vi "RangeSearch.vi"() -> ()   [LabVIEW 2019]
panel:
  in  "Start":bool
  in  "File Type":bool
  in  "stop":bool
  out "RPM Output":dbl
  out "Closest Range":dbl
  out "Array Index":dbl
  out "Search Value":dbl
  in  "Range":dbl(slide) scale=9.0..14.0
  out "Fractional Index":dbl
  out "Searched Part of 2D Array":dbl[](array[numeric])
  out "Input File":string
  out "Output Array":dbl[][](array[numeric])
  # "CSV Delimited"
  # "Tab Delimited"
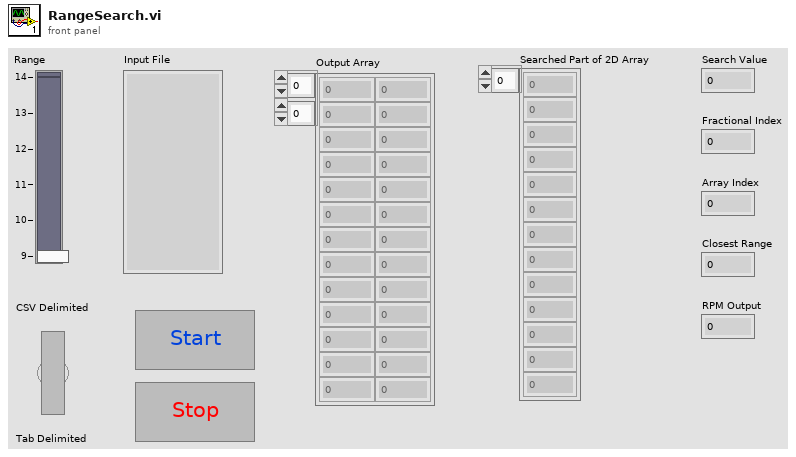
[diagram p1: front panel]
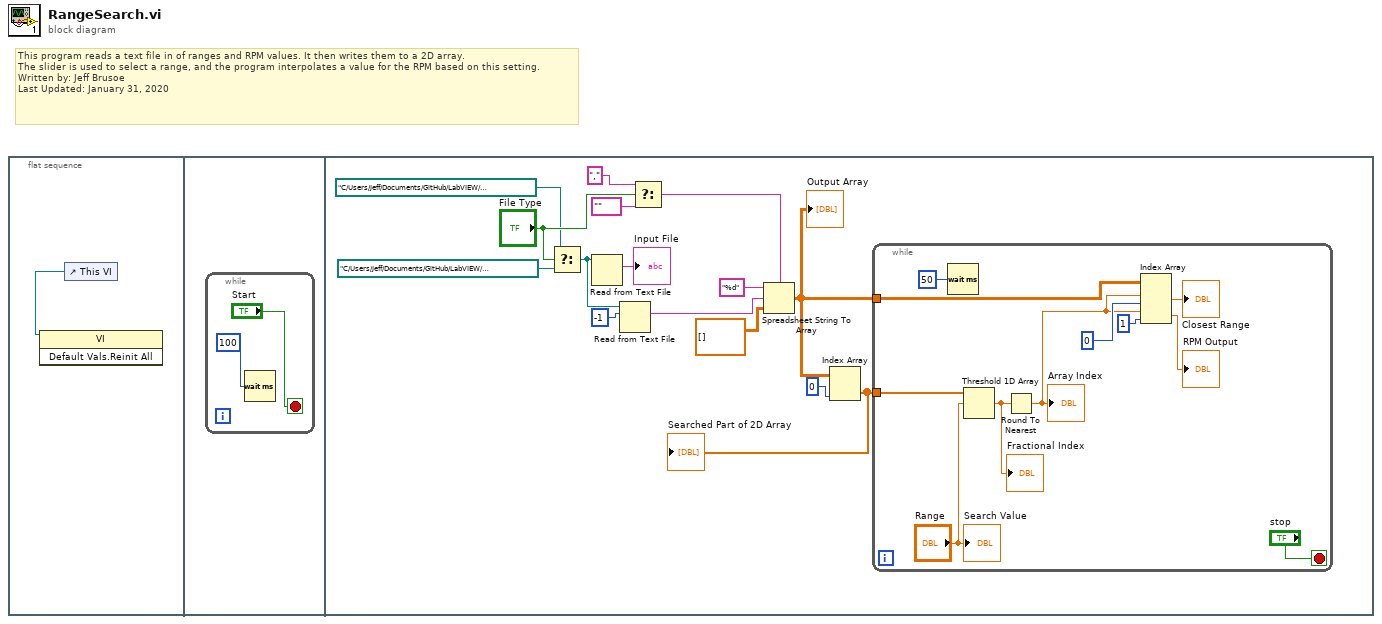
[diagram p0: block diagram]
diagram:
  # "This program reads a text file in of ranges and RPM values. It then writes them to a 2D array.\nThe slider is used to select a range, and the program interpolates a value for the RPM based on this setting.\nWritten by: Jeff Brusoe\nLast Updated: January 31, 2020"
  n1 = flat-sequence {
    frame #0 {
      n2 = control-ref of="This VI"() -> (w1:refnum<vi>)
      n3 = invoke class="VI" method="Default Vals.Reinit All"(reference=w1) -> ()  [unwired: 2 in, 3 out]
    }
    frame #1 {
      n4 = while {
        stop <- "Start" stop-if-true
        n5 = Wait (ms)(milliseconds to wait=u32 100) -> ()  [unwired: 1 out]
      }
    }
    frame #2 {
      n6 = Select(t=path "C:/Users/Jeff/Documents/GitHub/LabVIEW/3LabVIEWFeatures/RangeSearch/InputFileCSV.txt", s="File Type", f=path "C:/Users/Jeff/Documents/GitHub/LabVIEW/3LabVIEWFeatures/RangeSearch/InputFileTab.txt") -> (s? t:f=w17:path)
      n7 = Read from Text File(file (use dialog)=w17) -> (text=→"Input File":string)  [unwired: 3 in, 3 out]
      n8 = Read from Text File(file (use dialog)=w17, count=-1) -> (text=w12:string)  [unwired: 2 in, 3 out]
      n9 = Select(t=",", s="File Type", f="" ("format string")) -> (s? t:f=w18:string)
      n10 = Spreadsheet String To Array(delimiter (Tab)=w18, format string="%d", spreadsheet string=w12, array type (2D Dbl)=dbl[][] []) -> (array=w15:dbl[][])
      "Output Array" <- w15
      n11 = Index Array(array=w15, index (col)=0 ("disabled index (col)")) -> (element=w14:dbl[])  [unwired: 1 in]
      "Searched Part of 2D Array" <- w14
      n12 = while {
        tunnel: w14 -> [w29]
        tunnel: w15 -> [w24]
        stop <- "stop" stop-if-true
        n13 = Wait (ms)(milliseconds to wait=u32 50) -> ()  [unwired: 1 out]
        n14 = Threshold 1D Array(2:"Range", 3:w29) -> (0:w25:dbl)  [unwired: 1 in]
        "Fractional Index" <- w25
        n15 = Round To Nearest(number=w25) -> (nearest integer value=w20:dbl)
        "Array Index" <- w20
        n16 = Index Array(array=w24, index (row) #1=w20, index (col) #1=0 ("disabled index (col)"), index (row) #2=w20, index (col) #2=1 ("index (col)")) -> (element #1=→"Closest Range":dbl, element #2=→"RPM Output":dbl)
        "Search Value" <- "Range"
      }
    }
  }
